vi "M9347 phase.vi"(7 "Chan":u16(ring)=1 items=["Channel 2"=2, "Channel 1"=1], 8 "error in (no error)":errorcluster, 11 "Phase degree":dbl format="%#.4f") -> (0 "error out":errorcluster)   [LabVIEW 2023]
panel:
  in  "VISA resource name":refnum<visa-resource-name>="TCPIP0::localhost::hislip1::INSTR"
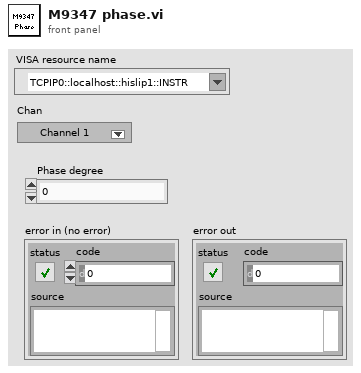
[diagram p1: front panel]
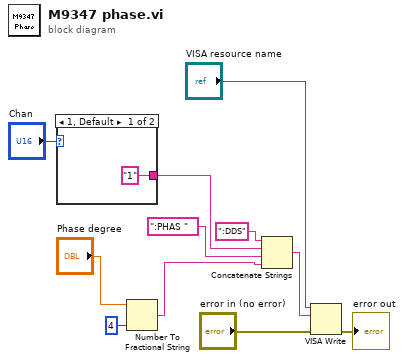
[diagram p0: block diagram]
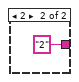
[diagram p2: hidden frame]
diagram:
  n1 = case shown="1, Default" "Chan" {
    tunnel: ["1" "2"] -> w9
    frame 1, Default {
    }
    frame 2 {
    }
  }
  n2 = Number To Fractional String(number="Phase degree", precision (6)=i16 4) -> (F-format string=w2:string)  [unwired: 2 in]
  n3 = Concatenate Strings(":DDS" ("string"), w9, ":PHAS " ("string"), w2) -> (w6:string)
  n4 = VISA Write(VISA resource name="VISA resource name", write buffer=w6, error in (no error)="error in (no error)") -> (error out=→"error out":errorcluster)  [unwired: 2 out]
